vi "Integral.vi"(1 "sum[k-1]":dbl, 2 "Ts":dbl, 3 "error":dbl) -> (0 "sum":dbl)   [LabVIEW 2011]
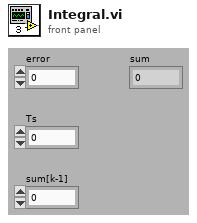
[diagram p1: front panel]
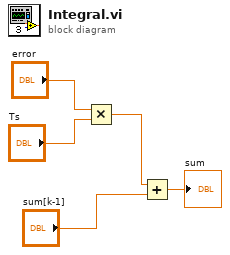
[diagram p0: block diagram]
diagram:
  n1 = Multiply(x="error", y="Ts") -> (x*y=w3:dbl)
  n2 = Add(x=w3, y="sum[k-1]") -> (x+y=→"sum":dbl)
